vi "Sweep.vi"() -> ()   [LabVIEW 2018]
uses:
  SesWrapper/SesWrapper.lvlib
panel:
  out "Library Information":string
  in  "Exit Button":bool
  in  "Working Directory":string="D:\\SES_1.9.0-beta.43_Win64"
  in  "Instrument Configuration File":string
  in  "Open Instrument":bool
  in  "Analyzer Region":T1={"fixed_"=0, "highEnergy_"=11.0, "lowEnergy_"=10.0, "centerEnergy_"=10.5, "energyStep_"=0.1, "dwellTime_"=200}
  in  "Detector Region":T2={"firstXChannel_"=1, "lastXChannel_"=800, "firstYChannel_"=1, "lastYChannel_"=649, "slices_"=1, "adcMode_"=1}
  in  "Element Set":string(combo)
  in  "Lens Mode":string(combo)
  in  "Pass Energy":string(combo)
  in  "Start Button":bool
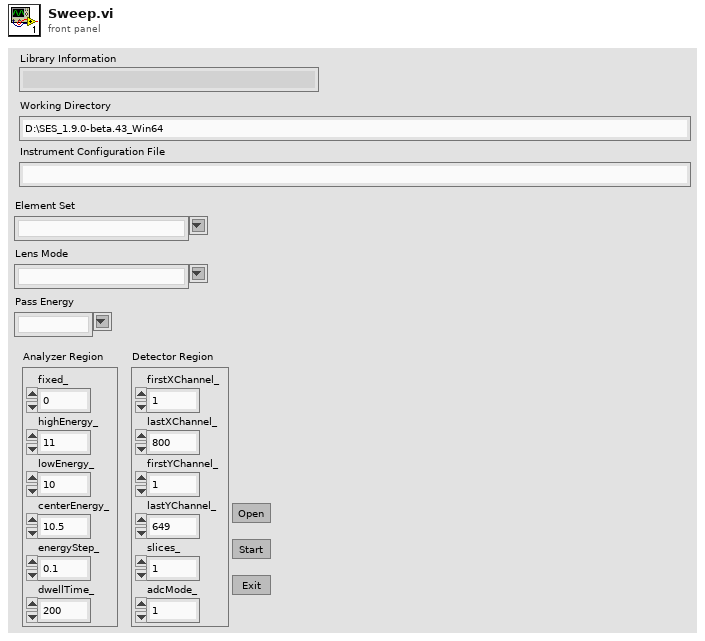
[diagram p1: front panel]
types:
  T1 = cluster{"fixed_":u8, "highEnergy_":dbl, "lowEnergy_":dbl, "centerEnergy_":dbl, "energyStep_":dbl, "dwellTime_":i32}
  T2 = cluster{"firstXChannel_":i32, "lastXChannel_":i32, "firstYChannel_":i32, "lastYChannel_":i32, "slices_":i32, "adcMode_":u8}
  T3 = cluster{"timerControlled_":u8, "@dummy control@":i8, "@dummy control@":i8, "@dummy control@":i8, "xChannels_":i32, "yChannels_":i32, "maxSlices_":i32, "maxChannels_":i32, "frameRate_":i32, "adcPresent_":u8, "discPresent_":u8}
  T4 = cluster{"timerControlled_":u8, "xChannels_":i32, "yChannels_":i32, "maxSlices_":i32, "maxChannels_":i32, "frameRate_":i32, "adcPresent_":u8, "discPresent_":u8}
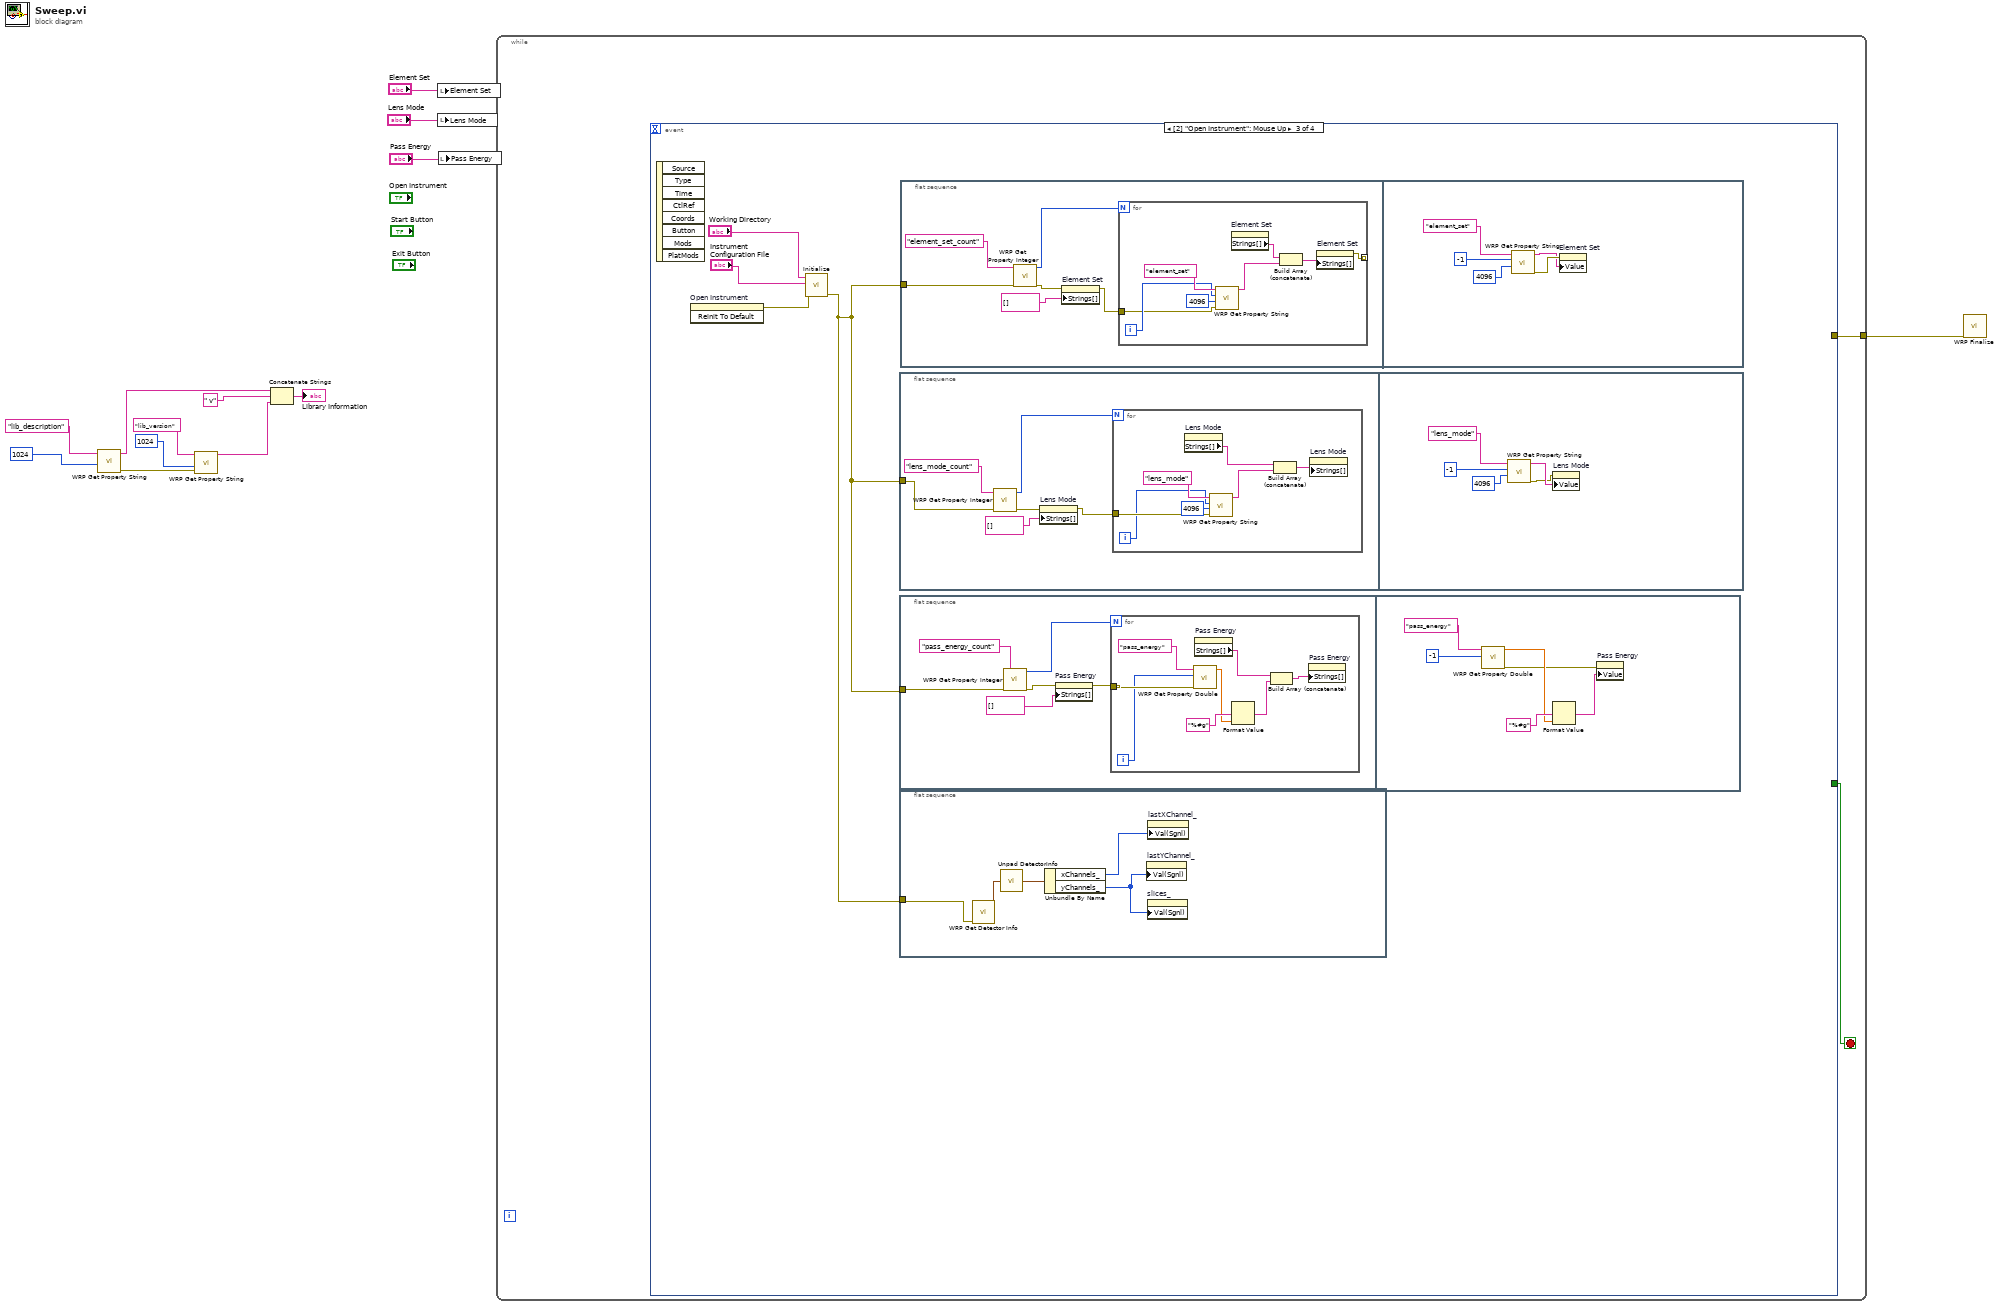
[diagram p0: block diagram]
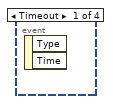
[diagram p2: hidden frame]
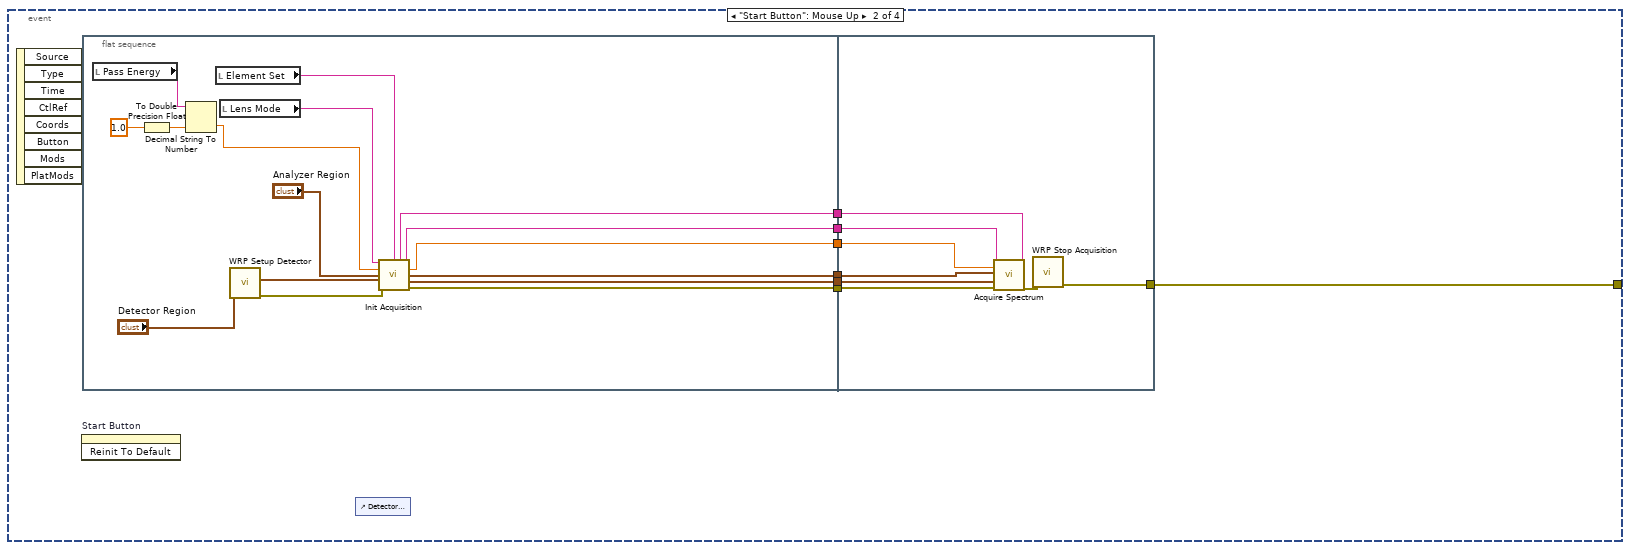
[diagram p3: hidden frame]
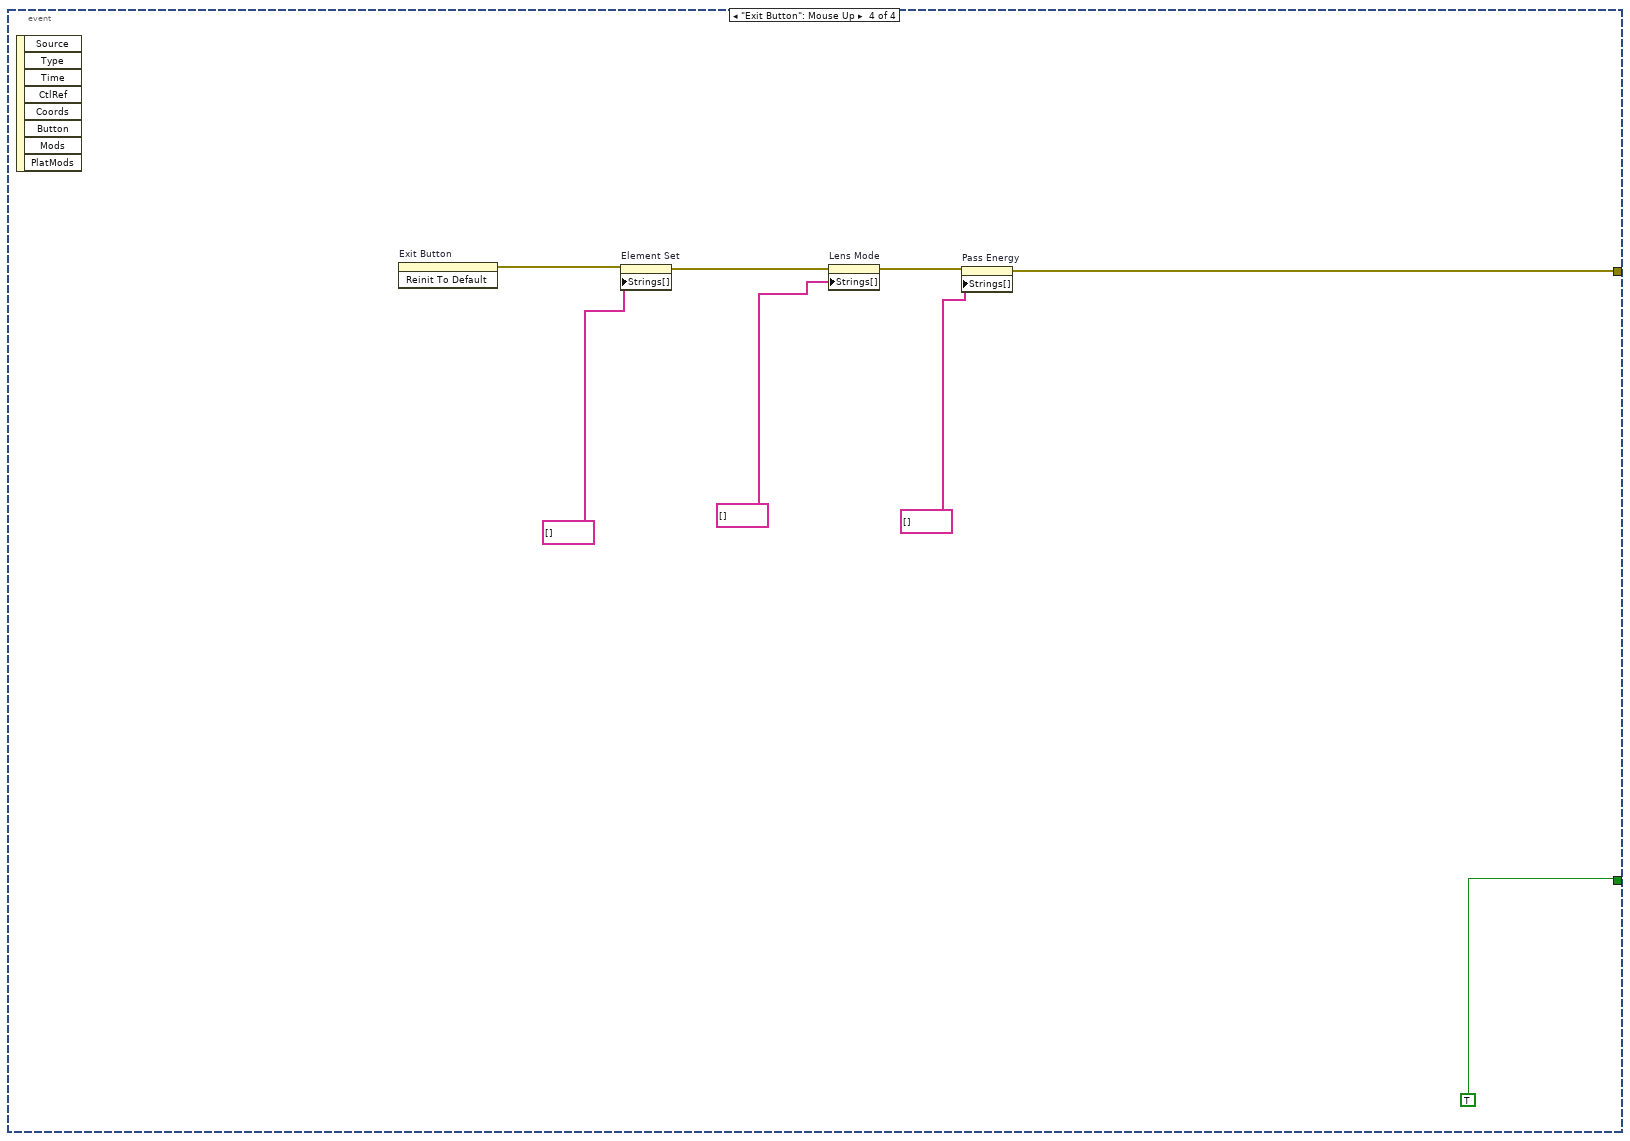
[diagram p4: hidden frame]
diagram:
  n1 = call "WRP Get Property String.vi"("size"=1024, "property"="lib_description") -> ("error out"=w7:errorcluster, "value"=w3:string)  [unwired: 6 in, 2 out]
  n2 = call "WRP Get Property String.vi"("error in (no error)"=w7, "size"=1024, "property"="lib_version") -> ("value"=w2:string)  [unwired: 5 in, 3 out]
  n3 = Concatenate Strings(w3, " v" ("string"), w2) -> (→"Library Information":string)
  n4 = local write "Element Set"("Element Set") -> ()
  n5 = local write "Lens Mode"("Lens Mode") -> ()
  n6 = local write "Pass Energy"("Pass Energy") -> ()
  n7 = while {
    tunnel: [w15] -> w10
    stop <- w14 stop-if-true
    n8 = event shown="[2] \"Open Instrument\": Mouse Up" {
      selector: _ -> [_ _ _ _]
      dyn-events: _ -> [_ _ _ _]
      timeout: _ -> [_ _ _ _]
      tunnel: [_ w20 _ w120] -> w15
      tunnel: [_ _ _ TRUE] -> w14
      event Timeout {
        n9 = event-data() -> ()  [unwired: 1 in, 2 out]
      }
      event "Start Button": Mouse Up {
        n10 = event-data() -> ()  [unwired: 1 in, 8 out]
        n11 = invoke on="Start Button" class="Bool" method="Reinit To Default"() -> ()  [unwired: 3 in, 3 out]
        n12 = flat-sequence {
          tunnel: [w37] -> w22
          tunnel: [w36] -> w21
          tunnel: [w29] -> w19
          tunnel: [w28] -> w18
          tunnel: [w24] -> w17
          tunnel: [w23] -> w16
          tunnel: w22 -> [w45]
          tunnel: w21 -> [w44]
          tunnel: [w43] -> w20
          tunnel: w19 -> [w42]
          tunnel: w18 -> [w41]
          tunnel: w17 -> [w40]
          tunnel: w16 -> [w39]
          frame #0 {
            n13 = local read "Pass Energy"() -> (w30:string)
            n14 = To Double Precision Float(number=1.0) -> (double precision float=w34:dbl)
            n15 = Decimal String To Number(string=w30, default (0L)=w34) -> (number=w35:dbl)  [unwired: 1 in, 1 out]
            n16 = local read "Element Set"() -> (w32:string)
            n17 = local read "Lens Mode"() -> (w31:string)
            n18 = call "WRP Setup Detector.vi"("detectorRegion"="Detector Region") -> ("error out"=w25:errorcluster, "detectorRegionOut"=w26:T2)  [unwired: 8 in, 1 out]
            n19 = call "Init Acquisition.vi"("Lens Mode"=w31, "element_set"=w32, "Pass Energy"=w35, "Region"="Analyzer Region", "Detector Region"=w26, "error in (no error)"=w25) -> ("element_set out"=w29:string, "Lens Mode out"=w37:string, "Pass Energy out"=w36:dbl, "Region out"=w28:T1, "Detector Region out"=w23:T2, "error out"=w24:errorcluster)  [unwired: 4 in]
          }
          frame #1 {
            n20 = call "Acquire Spectrum.vi"("Lens Mode"=w45, "Pass Energy"=w44, "Region"=w41, "Detector Region"=w39, "error in"=w40, "Element Set"=w42) -> ("error out"=w46:errorcluster)  [unwired: 13 in]
            n21 = call "WRP Stop Acquisition.vi"("error in (no error)"=w46) -> ("error out"=w43:errorcluster)  [unwired: 9 in, 1 out]
          }
        }
        n22 = control-ref of="Detector Region"() -> ()  [unwired: 1 out]
      }
      event "Open Instrument": Mouse Up {
        n23 = event-data() -> ()  [unwired: 1 in, 8 out]
        n24 = invoke on="Open Instrument" class="Bool" method="Reinit To Default"() -> (error out=w49:errorcluster)  [unwired: 3 in, 2 out]
        n25 = call "Initialize.vi"("error in (no error)"=w49, "Instrument Configuration File"="Instrument Configuration File", "working_directory"="Working Directory") -> ("error out"=w47:errorcluster)  [unwired: 8 in]
        n26 = flat-sequence {
          tunnel: w47 -> [w76]
          frame #0 {
            n27 = call "WRP Get Property Integer.vi"("error in (no error)"=w76, "property"="lens_mode_count") -> ("error out"=w78:errorcluster, "value"=w80:i32)  [unwired: 6 in, 2 out]
            n28 = property on="Lens Mode" class="CmbBox"(error in=w78, "Strings[]"=string[] [] ("Strings []")) -> (error out=w81:errorcluster)  [unwired: 1 in, 1 out]
            n29 = for {
              N: w80 -> [_]
              tunnel: w81 -> [w87]
              i -> [w85]
              n30 = property on="Lens Mode" class="CmbBox"() -> ("Strings[]"=w83:string[])  [unwired: 2 in, 2 out]
              n31 = call "WRP Get Property String.vi"("error in (no error)"=w87, "size"=4096, "index"=w85, "property"="lens_mode") -> ("value"=w84:string)  [unwired: 4 in, 3 out]
              n32 = Build Array (concatenate)(w83, w84) -> (w82:string[])
              n33 = property on="Lens Mode" class="CmbBox"("Strings[]"=w82) -> ()  [unwired: 2 in, 2 out]
            }
          }
          frame #1 {
            n34 = call "WRP Get Property String.vi"("size"=4096, "index"=-1, "property"="lens_mode") -> ("error out"=w90:errorcluster, "value"=w91:string)  [unwired: 5 in, 2 out]
            n35 = property on="Lens Mode" class="CmbBox"(error in=w90, "Value"=w91) -> ()  [unwired: 1 in, 2 out]
          }
        }
        n36 = flat-sequence {
          tunnel: w47 -> [w56]
          frame #0 {
            n37 = call "WRP Get Property Integer.vi"("error in (no error)"=w56, "property"="pass_energy_count") -> ("error out"=w60:errorcluster, "value"=w57:i32)  [unwired: 6 in, 2 out]
            n38 = property on="Pass Energy" class="CmbBox"(error in=w60, "Strings[]"=string[] [] ("Strings []")) -> (error out=w58:errorcluster)  [unwired: 1 in, 1 out]
            n39 = for {
              N: w57 -> [_]
              tunnel: w58 -> [w68]
              i -> [w65]
              n40 = call "WRP Get Property Double.vi"("error in (no error)"=w68, "index"=w65, "property"="pass_energy") -> ("value"=w62:dbl)  [unwired: 5 in, 3 out]
              n41 = property on="Pass Energy" class="CmbBox"() -> ("Strings[]"=w67:string[])  [unwired: 2 in, 2 out]
              n42 = Format Value(format string="%#g", value (0)=w62) -> (output string=w64:string)  [unwired: 1 in]
              n43 = Build Array (concatenate)(w67, w64) -> (w66:string[])
              n44 = property on="Pass Energy" class="CmbBox"("Strings[]"=w66) -> ()  [unwired: 2 in, 2 out]
            }
          }
          frame #1 {
            n45 = call "WRP Get Property Double.vi"("index"=-1, "property"="pass_energy") -> ("error out"=w70:errorcluster, "value"=w72:dbl)  [unwired: 6 in, 2 out]
            n46 = Format Value(format string="%#g", value (0)=w72) -> (output string=w71:string)  [unwired: 1 in]
            n47 = property on="Pass Energy" class="CmbBox"(error in=w70, "Value"=w71) -> ()  [unwired: 1 in, 2 out]
          }
        }
        n48 = flat-sequence {
          tunnel: w47 -> [w53]
          frame #0 {
            n49 = call "WRP Get Detector Info.vi"("error in (no error)"=w53) -> ("value"=w54:T3)  [unwired: 8 in, 2 out]
            n50 = call "Unpad DetectorInfo.vi"("Detector Info"=w54) -> ("Detector Info out"=w55:T4)
            n51 = Unbundle By Name(w55) -> ("xChannels_"=w52:i32, "yChannels_"=w51:i32)
            n52 = property on="lastYChannel_" class="DigNum (strict)"("Val(Sgnl)"=w51) -> ()  [unwired: 2 in, 2 out]
            n53 = property on="slices_" class="DigNum (strict)"("Val(Sgnl)"=w51) -> ()  [unwired: 2 in, 2 out]
            n54 = property on="lastXChannel_" class="DigNum (strict)"("Val(Sgnl)"=w52) -> ()  [unwired: 2 in, 2 out]
          }
        }
        n55 = flat-sequence {
          tunnel: w47 -> [w96]
          frame #0 {
            n56 = call "WRP Get Property Integer.vi"("error in (no error)"=w96, "property"="element_set_count") -> ("error out"=w95:errorcluster, "value"=w98:i32)  [unwired: 6 in, 2 out]
            n57 = property on="Element Set" class="CmbBox"(error in=w95, "Strings[]"=string[] [] ("Strings []")) -> (error out=w94:errorcluster)  [unwired: 1 in, 1 out]
            n58 = for {
              N: w98 -> [_]
              tunnel: [w101] -> _ mode=indexing
              tunnel: w94 -> [w100]
              i -> [w105]
              n59 = call "WRP Get Property String.vi"("error in (no error)"=w100, "size"=4096, "index"=w105, "property"="element_set") -> ("value"=w104:string)  [unwired: 4 in, 3 out]
              n60 = property on="Element Set" class="CmbBox"() -> ("Strings[]"=w102:string[])  [unwired: 2 in, 2 out]
              n61 = Build Array (concatenate)(w102, w104) -> (w103:string[])
              n62 = property on="Element Set" class="CmbBox"("Strings[]"=w103) -> (error out=w101:errorcluster)  [unwired: 2 in, 1 out]
            }
          }
          frame #1 {
            n63 = call "WRP Get Property String.vi"("size"=4096, "index"=-1, "property"="element_set") -> ("error out"=w110:errorcluster, "value"=w109:string)  [unwired: 5 in, 2 out]
            n64 = property on="Element Set" class="CmbBox"(error in=w110, "Value"=w109) -> ()  [unwired: 1 in, 2 out]
          }
        }
      }
      event "Exit Button": Mouse Up {
        n65 = event-data() -> ()  [unwired: 1 in, 8 out]
        n66 = invoke on="Exit Button" class="Bool" method="Reinit To Default"() -> (error out=w113:errorcluster)  [unwired: 3 in, 2 out]
        n67 = property on="Element Set" class="CmbBox"(error in=w113, "Strings[]"=string[] [] ("Strings []")) -> (error out=w119:errorcluster)  [unwired: 1 in, 1 out]
        n68 = property on="Lens Mode" class="CmbBox"(error in=w119, "Strings[]"=string[] [] ("Strings []")) -> (error out=w118:errorcluster)  [unwired: 1 in, 1 out]
        n69 = property on="Pass Energy" class="CmbBox"(error in=w118, "Strings[]"=string[] [] ("Strings []")) -> (error out=w120:errorcluster)  [unwired: 1 in, 1 out]
      }
    }
  }
  n70 = call "WRP Finalize.vi"("error in (no error)"=w10) -> ()  [unwired: 9 in, 2 out]
